vi "Update Table Value & Format.vi"(8 "error in (no error)":errorcluster, 11 "Text based Communications Test in":refnum<class "Text based Communications Test.lvclass">) -> (0 "error out":errorcluster, 3 "Text based Communications Test out":refnum<class "Text based Communications Test.lvclass">)   [LabVIEW 2017, in "Text based Communications Test.lvlib" / "Text based Communications Test.lvclass"]
uses:
  Text based Communications Test.lvclass
  <vilib>/Utility/miscctls.llb/LVRowAndColumnTypeDef.ctl
  Text based Communications Test.lvclass/Text based Communications Test.ctl
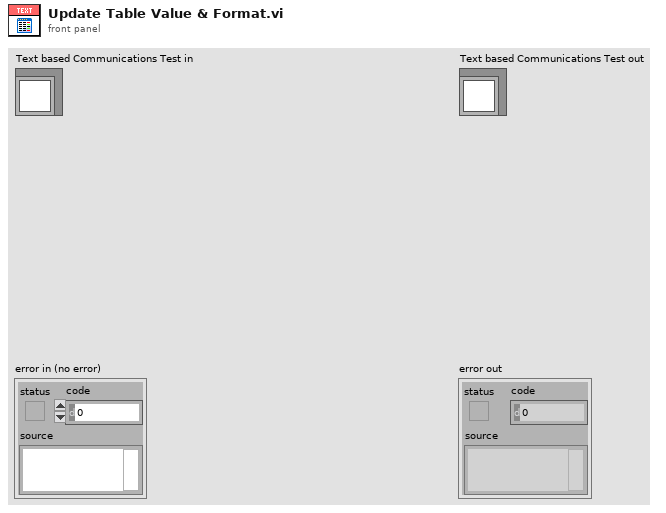
[diagram p1: front panel]
types:
  T1 = typedef "LVRowAndColumnTypeDef.ctl" = cluster{"Row":i32, "Column":i32}
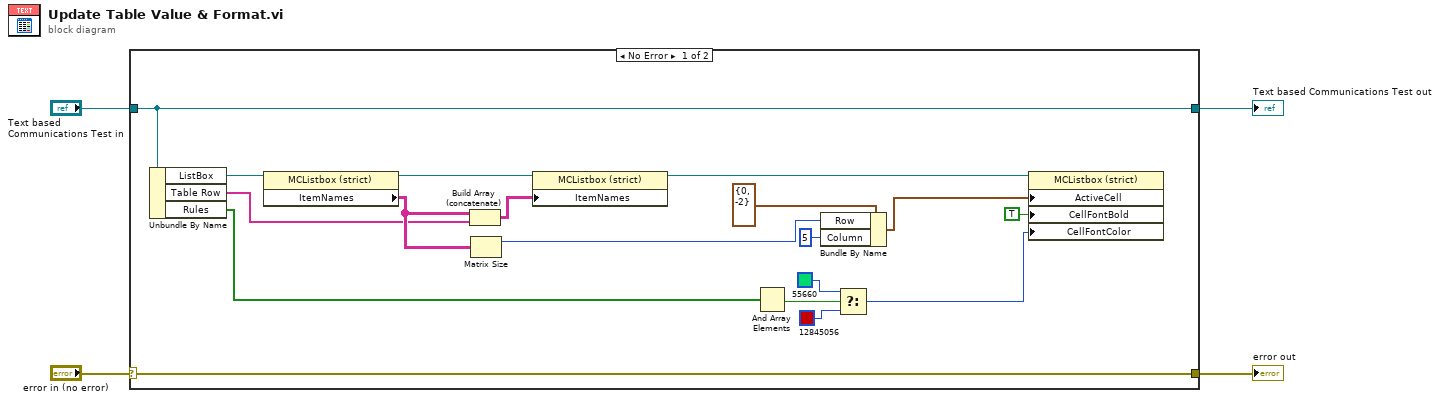
[diagram p0: block diagram]
diagram:
  n1 = case shown="No Error" "error in (no error)" {
    selector: "error in (no error)" -> [w22 w24]
    tunnel: [w22 w24] -> w3
    tunnel: [w21 w23] -> w1
    tunnel: "Text based Communications Test in" -> [w21 w23]
    frame No Error {
      n2 = Unbundle By Name(w21) -> ("ListBox"=w19:refnum<vi>, "Table Row"=w18:string[], "Rules"=w14:bool[])
      n3 = property class="MCListbox (strict)"(reference=w19) -> (reference out=w16:refnum<vi>, "ItemNames"=w20:string[][])  [unwired: 1 in, 1 out]
      n4 = Build Array (concatenate)(w20, w18) -> (w17:string[][])
      n5 = Matrix Size(0:w20) -> (1:w13:i32)  [unwired: 1 out]
      n6 = property class="MCListbox (strict)"(reference=w16, "ItemNames"=w17) -> (reference out=w6:refnum<vi>)  [unwired: 1 in, 1 out]
      n7 = And Array Elements(Boolean array=w14) -> (logical AND=w10:bool)
      n8 = Bundle By Name(cluster=T1 {"Row"=0, "Column"=-2} ("Active Cell:Active Cell"), "Row"=w13, "Column"=5) -> (w11:T1)
      n9 = Select(t=u32 55660 ("Color Box"), s=w10, f=u32 12845056 ("Color Box")) -> (s? t:f=w7:u32)
      n10 = property class="MCListbox (strict)"(reference=w6, "ActiveCell"=w11, "CellFontBold"=TRUE ("Active Cell:Cell Font:Bold"), "CellFontColor"=w7) -> ()  [unwired: 1 in, 2 out]
    }
    frame Error {
    }
  }
  "error out" <- w3
  "Text based Communications Test out" <- w1
